vi "CRYSpectrum Unit Conv dBref.vi"(4 "window constants":cluster{"eq noise BW":dbl, "coherent gain":dbl}={"eq noise BW"=1.0, "coherent gain"=1.0} {"coherent gain" format="%.2f"; "eq noise BW" format="%.2f"}, 5 "dB ref.":dbl format="%.2f", 6 "df":dbl=1.0 format="%.2f", 7 "signal unit (V)":string="V", 8 "display unit":T2(ring), 9 "log/linear":enum16{"Linear", "dB", "dBm"}(ring)=enum."dB", 10 "spectrum type":T1(ring), 11 "Spectrum":dbl[](array[numeric]) format="%.2f") -> (0 "spectrum unit":string="dBVrms", 3 "Spectrum":dbl[](array[numeric]) format="%.2f")   [LabVIEW 2013]
doc: "Converts the input spectrum (power, amplitude, or gain) to alternate formats including Log (dB or dBm) and spectral density.\n\nSpectrum is the input array containing a spectrum of the type specified by the spectrum type selector:\n spectrum type = 0 Power (Vrms^2)\n spectrum type = 1 Amplitude (Vrms)\n spectrum type = 2 Gain (amplitude ratio)\n\nThe signal unit (V) string control specifies the units of the spectrum. The signal unit (V) control defaults to V (volts).\n\nThe log/linear control has three selections for the output unit type\n log/linear = 0 Linear\n log/linear = 1 dB\n log/linear = 2 dBm\n\nThe display unit has the following selections for the display unit:\n 0: Vrms (volts rms)\n 1: Vpk (volts peak)\n 2: Vrms^2 (volts squared rms)\n 3: Vpk^2 (volts squared peak)\n 4: Vrms/ÃHz (volts rms per root Hz)\n 5: Vpk/ÃHz (volts peak per root Hz)\n 6: Vrms^2/Hz (volts squared rms per Hz)\n 7: Vpk^2/Hz (volts squared peak per Hz)\n\nThe last four selections are amplitude spectral density (4,5) and power spectral density (6,7).\nThe control cluster window constants contains constants for the selected window (from the Scaled Time Domain Window VI). You need this input only when you use the spectral density output formats (the last four output unit selections)."
panel:
  # "Spectrum Unit Conversion"
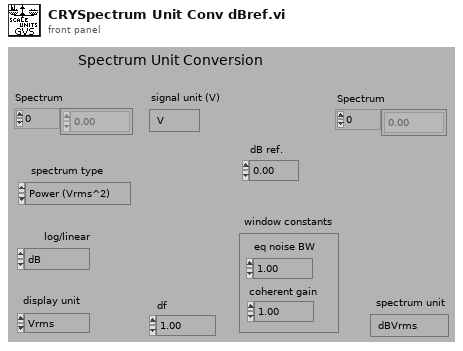
[diagram p1: front panel]
types:
  T1 = enum16{"Power (Vrms^2)", "Amplitude (Vrms)", "Gain (amplitude ratio)"}
  T2 = enum32{"Vrms", "Vpk", "Vrms^2", "Vpk^2", "Vrms/rtHz", "Vpk/rtHz", "Vrms^2/Hz", "Vpk^2/Hz"}
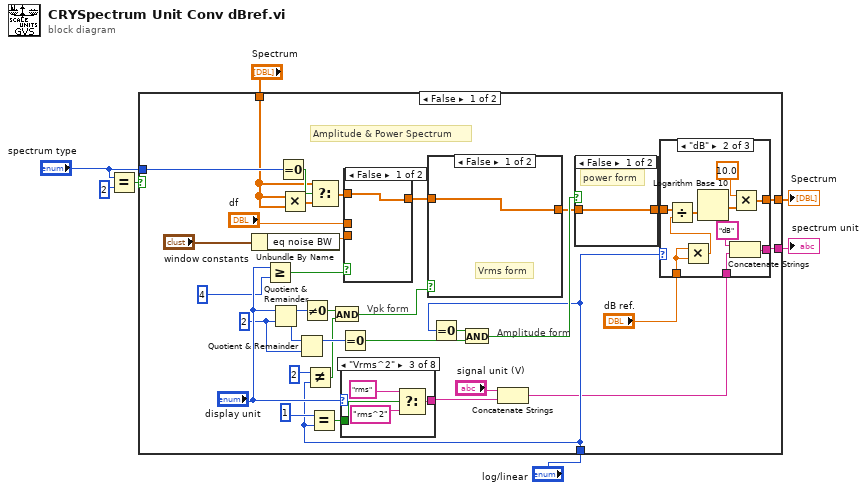
[diagram p0: block diagram]
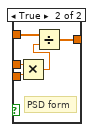
[diagram p2: hidden frame]
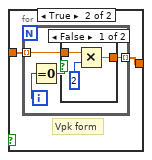
[diagram p3: hidden frame]
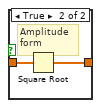
[diagram p5: hidden frame]
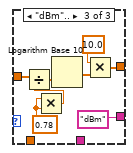
[diagram p7: hidden frame]
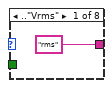
[diagram p8: hidden frame]
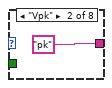
[diagram p9: hidden frame]
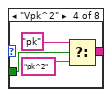
[diagram p10: hidden frame]
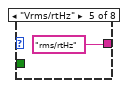
[diagram p11: hidden frame]
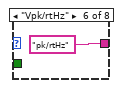
[diagram p12: hidden frame]
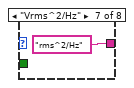
[diagram p13: hidden frame]
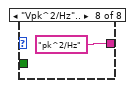
[diagram p14: hidden frame]
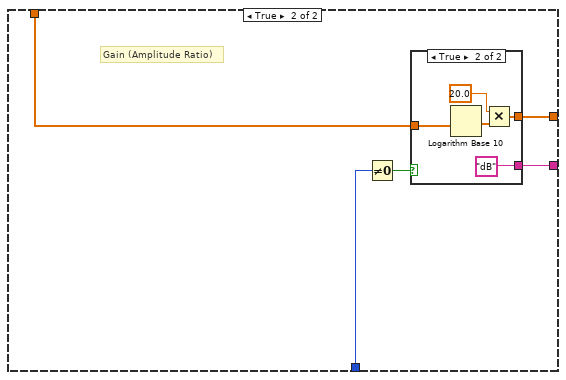
[diagram p15: hidden frame]
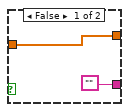
[diagram p16: hidden frame]
diagram:
  n1 = Equal?(x="spectrum type", y=2) -> (x = y?=w6:bool)
  n2 = case shown="False" w6 {
    tunnel: [w24 w100] -> w7
    tunnel: [w23 w99] -> w1
    tunnel: "spectrum type" -> [w21 _]
    tunnel: "Spectrum" -> [w20 w98]
    tunnel: "log/linear" -> [w15 w96]
    frame False {
      w35 = 2
      # "Amplitude & Power Spectrum"
      # "Vpk form"
      # "Amplitude form"
      n3 = Unbundle By Name("window constants") -> ("eq noise BW"=w31:dbl)
      n4 = Greater Or Equal?(x="display unit", y=4) -> (x >= y?=w28:bool)
      n5 = Quotient & Remainder(x="display unit", y=w35) -> (x-y*floor(x/y)=w32:u32, floor(x/y)=w34:u32)
      n6 = Equal To 0?(x=w21) -> (x = 0?=w25:bool)
      n7 = Multiply(x=w20, y=w20) -> (x*y=w26:dbl[])
      n8 = Quotient & Remainder(x=w34, y=w35) -> (x-y*floor(x/y)=w36:u32)  [unwired: 1 out]
      n9 = Not Equal To 0?(x=w32) -> (x != 0?=w13:bool)
      n10 = Not Equal?(x=2, y=w15) -> (x != y?=w14:bool)
      n11 = Equal?(x=1, y=w15) -> (x = y?=w18:bool)
      n12 = Select(t=w20, s=w25, f=w26) -> (s? t:f=w29:dbl[])
      n13 = And(x=w13, y=w14) -> (x .and. y?=w12:bool)
      n14 = Equal To 0?(x=w36) -> (x = 0?=w17:bool)
      n15 = case shown="\"Vrms^2\"" "display unit" {
        tunnel: ["rms" "pk" w87 w91 "rms/rtHz" "pk/rtHz" "rms^2/Hz" "pk^2/Hz"] -> w10
        tunnel: w18 -> [_ _ w86 w90 _ _ _ _]
        frame .."Vrms" {
        }
        frame "Vpk" {
        }
        frame "Vrms^2" {
          n16 = Select(t="rms", s=w86, f="rms^2") -> (s? t:f=w87:string)
        }
        frame "Vpk^2" {
          n17 = Select(t="pk", s=w90, f="pk^2") -> (s? t:f=w91:string)
        }
        frame "Vrms/rtHz" {
        }
        frame "Vpk/rtHz" {
        }
        frame "Vrms^2/Hz" {
        }
        frame "Vpk^2/Hz".. {
        }
      }
      n18 = case shown="False" w28 {
        tunnel: [w42 w46] -> w33
        tunnel: w31 -> [_ w45]
        tunnel: w29 -> [w42 w47]
        tunnel: "df" -> [_ w44]
        frame False {
        }
        frame True {
          # "PSD form"
          n19 = Multiply(x=w44, y=w45) -> (x*y=w43:dbl)
          n20 = Divide(x=w47, y=w43) -> (x/y=w46:dbl[])
        }
      }
      n21 = case shown="False" w12 {
        tunnel: [w48 w49] -> w37
        tunnel: w33 -> [w48 w50]
        frame False {
          # "Vrms form"
        }
        frame True {
          # "Vpk form"
          n22 = for {
            tunnel: [w51] -> w49 mode=indexing
            tunnel: w50 -> [w52] mode=indexing
            i -> [w54]
            n23 = Equal To 0?(x=w54) -> (x = 0?=w53:bool)
            n24 = case shown="False" w53 {
              tunnel: [w55 w58] -> w51
              tunnel: w52 -> [w57 w58]
              frame False {
                n25 = Multiply(x=w57, y=2) -> (x*y=w55:dbl)
              }
              frame True {
              }
            }
          }
        }
      }
      n26 = Equal To 0?(x=w15) -> (x = 0?=w41:bool)
      n27 = And(x=w41, y=w17) -> (x .and. y?=w40:bool)
      n28 = Concatenate Strings("signal unit (V)", w10) -> (w9:string)
      n29 = case shown="False" w40 {
        tunnel: [w59 w60] -> w38
        tunnel: w37 -> [w59 w61]
        frame False {
          # "power form"
        }
        frame True {
          # "Amplitude \nform"
          n30 = Square Root(x=w61) -> (sqrt(x)=w60:dbl[])
        }
      }
      n31 = case shown="\"dB\"" w15 {
        tunnel: w38 -> [w62 w65 w77]
        tunnel: w9 -> [w63 w70 _]
        tunnel: [w63 w69 "dBm"] -> w23
        tunnel: [w62 w68 w79] -> w24
        tunnel: "dB ref." -> [_ w67 _]
        frame .."Linear" {
        }
        frame "dB" {
          n32 = Multiply(x=w67, y=w67) -> (x*y=w66:dbl)
          n33 = Divide(x=w65, y=w66) -> (x/y=w64:dbl[])
          n34 = Logarithm Base 10(1:w64) -> (0:w73:dbl[])
          n35 = Concatenate Strings("dB", w70) -> (w69:string)
          n36 = Multiply(x=10.0, y=w73) -> (x*y=w68:dbl[])
        }
        frame "dBm".. {
          w75 = 0.78
          n37 = Multiply(x=w75, y=w75) -> (x*y=w74:dbl)
          n38 = Divide(x=w77, y=w74) -> (x/y=w78:dbl[])
          n39 = Logarithm Base 10(1:w78) -> (0:w81:dbl[])
          n40 = Multiply(x=10.0, y=w81) -> (x*y=w79:dbl[])
        }
      }
    }
    frame True {
      # "Gain (Amplitude Ratio)"
      n41 = Not Equal To 0?(x=w96) -> (x != 0?=w97:bool)
      n42 = case shown="True" w97 {
        tunnel: [w102 w103] -> w100
        tunnel: w98 -> [w102 w107]
        tunnel: ["" "dB"] -> w99
        frame False {
        }
        frame True {
          n43 = Logarithm Base 10(1:w107) -> (0:w106:dbl[])
          n44 = Multiply(x=20.0, y=w106) -> (x*y=w103:dbl[])
        }
      }
    }
  }
  "spectrum unit" <- w1
  "Spectrum" <- w7
